vi "Write Total Rect.vi"(5 "Total Rect":T1, 9 "GObject in":refnum<class "GObject.lvclass">) -> (3 "GObject out":refnum<class "GObject.lvclass">)   [LabVIEW 2014, in "GObject.lvclass"]
uses:
  GObject.lvclass
  <vilib>/Utility/miscctls.llb/LVRectTypeDef.ctl
  GObject.lvclass/GObject.ctl
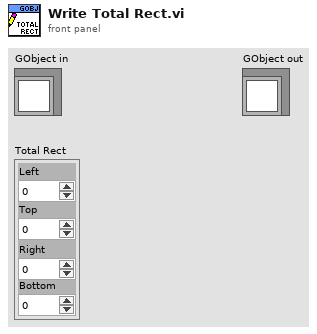
[diagram p1: front panel]
types:
  T1 = typedef "LVRectTypeDef.ctl" = cluster{"Left":i16, "Top":i16, "Right":i16, "Bottom":i16}
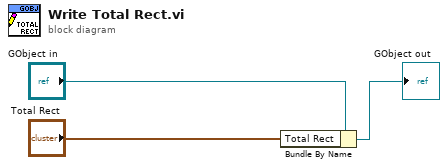
[diagram p0: block diagram]
diagram:
  n1 = Bundle By Name(cluster="GObject in", "Total Rect"="Total Rect") -> (→"GObject out":refnum<class "GObject.lvclass">)
